vi "FGV SapID.vi"(10 "Enum":enum16{"write", "read"}(ring)=enum."read", 11 "SapID":u16) -> (3 "SapID":u16)   [LabVIEW 2018, in "Application.lvlib"]
uses:
  Application/Application.lvlib
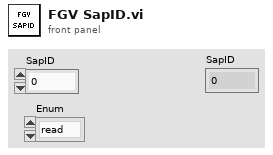
[diagram p1: front panel]
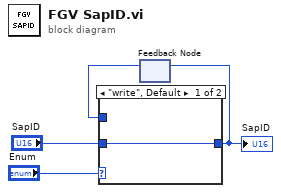
[diagram p0: block diagram]
diagram:
  n1 = feedback #1() -> (w3:u16)  [unwired: 1 in]
  n2 = case shown="\"write\", Default" "Enum" {
    tunnel: w3 -> [_ w6]
    tunnel: [w5 w6] -> w2
    tunnel: "SapID" -> [w5 _]
    frame "write", Default {
    }
    frame "read" {
    }
  }
  "SapID" <- w2
  n3 = feedback-in #1(w2) -> ()
